vi "iX2 v1.0.vi"(1 "On_Off":bool=TRUE, 2 "Input":dbl min=-1.0 max=1.0 step=0.05) -> (8 "s? t:f":dbl)   [LabVIEW 2014]
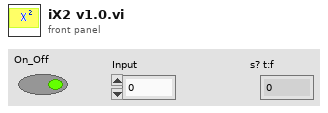
[diagram p1: front panel]
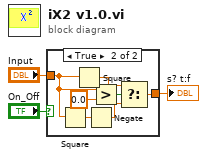
[diagram p0: block diagram]
diagram:
  n1 = case shown="True" "On_Off" {
    tunnel: "Input" -> [w4 w6]
    tunnel: [w4 w5] -> w2
    frame False {
    }
    frame True {
      n2 = Square(x=w6) -> (x^2=w8:dbl)
      n3 = Square(x=w6) -> (x^2=w9:dbl)
      n4 = Negate(x=w8) -> (-x=w7:dbl)
      n5 = Greater?(x=w6, y=0.0) -> (0:w11:bool)
      n6 = Select(t=w9, s=w11, f=w7) -> (s? t:f=w5:dbl)
    }
  }
  "s? t:f" <- w2
